vi "SSC DAQmx Read TEDS.vi"(0 "DAQmx SSC in":T2[](array[typedef]), 11 "error in":errorcluster) -> (4 "DAQmx SSC out":T2[](array[typedef]), 6 "SSC TEDS BitStream":T1[][](array[typedef]), 15 "error out":errorcluster)   [LabVIEW 2020]
doc: "Reads the TEDS bitstream in the order of SSC."
uses:
  Pin Map/SSC DAQmx.ctl
  Typedefs/SSC TEDS Bitstream.ctl
  <resource>/objmgr/daqmx.rc
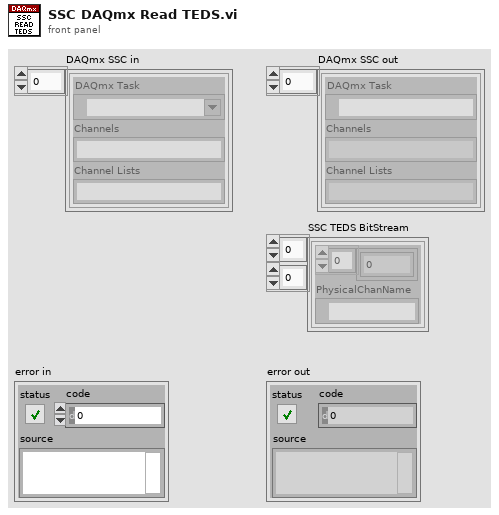
[diagram p1: front panel]
types:
  T1 = typedef "SSC TEDS Bitstream.ctl" = cluster{"TEDS BitStream":u8[], "PhysicalChanName":tag}
  T2 = typedef "SSC DAQmx.ctl" = cluster{"DAQmx Task ":refnum<k21>, "Channels":string, "Channel Lists":string}
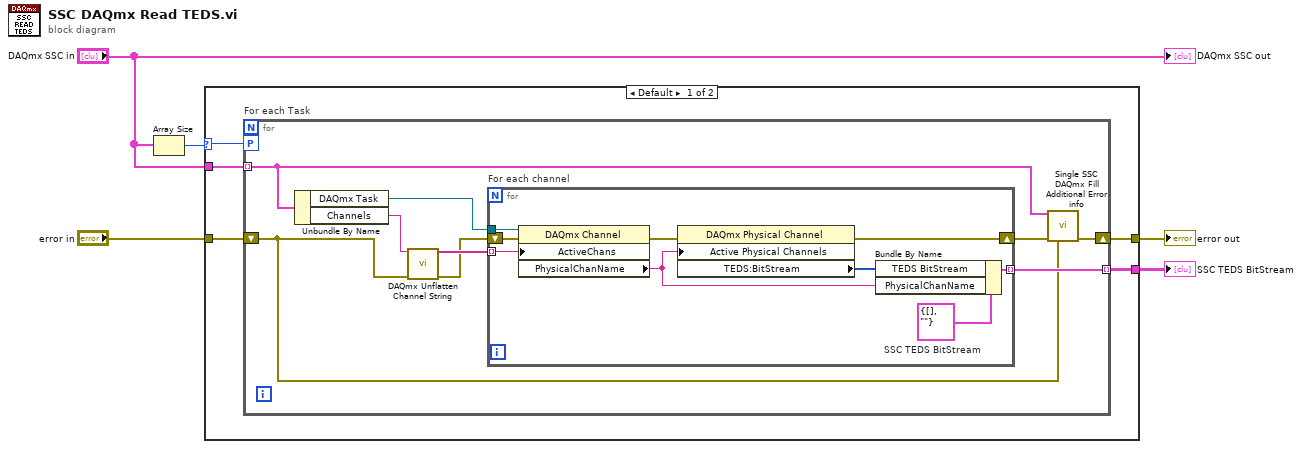
[diagram p0: block diagram]
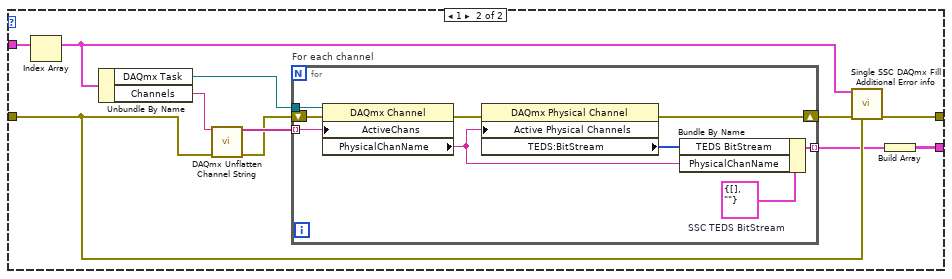
[diagram p2: hidden frame]
diagram:
  n1 = Array Size(array="DAQmx SSC in") -> (size(s)=w3:i32)
  n2 = case shown="Default" w3 {
    selector: w3 -> [w8 _]
    tunnel: [w10 w39] -> w5
    tunnel: "error in" -> [w9 w38]
    tunnel: "DAQmx SSC in" -> [w7 w37]
    tunnel: [w6 w29] -> w1
    frame Default {
      n3 = for "For each Task" {
        tunnel: w7 -> [w18] mode=indexing
        workers-P: w8 -> [_]
        shift-right: [w19] -> w10
        shift-left: w9 -> [w12]
        tunnel: [w15] -> w6 mode=indexing
        n4 = Unbundle By Name(w18) -> ("DAQmx Task"=w16:refnum<k21>, "Channels"=w14:string)
        n5 = call <vilib>:"DAQmx Unflatten Channel String.vi"("names in"=w14, "error in"=w12) -> ("names out"=w13:string[], "error out"=w11:errorcluster)  [unwired: 12 in]
        n6 = for "For each channel" {
          shift-right: [w28] -> w17
          shift-left: w11 -> [w27]
          tunnel: w16 -> [w25]
          tunnel: w13 -> [w24] mode=indexing
          tunnel: [w22] -> w15 mode=indexing
          w23 = T1 {"TEDS BitStream"=[], "PhysicalChanName"=""}  # SSC TEDS BitStream
          n7 = property class="DAQmx Channel"(reference=w25, error in=w27, "ActiveChans"=w24) -> (error out=w26:errorcluster, "PhysicalChanName"=w20:tag)  [unwired: 1 out]
          n8 = property class="DAQmx Physical Channel"(error in=w26, "Active Physical Channels"=w20) -> (error out=w28:errorcluster, "TEDS:BitStream"=w21:u8[])  [unwired: 1 in, 1 out]
          n9 = Bundle By Name(cluster=w23, "TEDS BitStream"=w21, "PhysicalChanName"=w20) -> (w22:T1)
        }
        n10 = call "Single SSC DAQmx Fill Additional Error info.vi"("DAQmx SSC in"=w18, "error in"=w17, "previous error in"=w12) -> ("error out"=w19:errorcluster)  [unwired: 12 in]
      }
    }
    frame 1 {
      n11 = Index Array(array=w37) -> (element=w30:T2)  [unwired: 1 in]
      n12 = Unbundle By Name(w30) -> ("DAQmx Task"=w34:refnum<k21>, "Channels"=w33:string)
      n13 = call <vilib>:"DAQmx Unflatten Channel String.vi"("names in"=w33, "error in"=w38) -> ("names out"=w32:string[], "error out"=w31:errorcluster)  [unwired: 12 in]
      n14 = for "For each channel" {
        shift-right: [w48] -> w35
        shift-left: w31 -> [w47]
        tunnel: w34 -> [w45]
        tunnel: w32 -> [w44] mode=indexing
        tunnel: [w42] -> w36 mode=indexing
        w43 = T1 {"TEDS BitStream"=[], "PhysicalChanName"=""}  # SSC TEDS BitStream
        n15 = property class="DAQmx Channel"(reference=w45, error in=w47, "ActiveChans"=w44) -> (error out=w46:errorcluster, "PhysicalChanName"=w40:tag)  [unwired: 1 out]
        n16 = property class="DAQmx Physical Channel"(error in=w46, "Active Physical Channels"=w40) -> (error out=w48:errorcluster, "TEDS:BitStream"=w41:u8[])  [unwired: 1 in, 1 out]
        n17 = Bundle By Name(cluster=w43, "TEDS BitStream"=w41, "PhysicalChanName"=w40) -> (w42:T1)
      }
      n18 = call "Single SSC DAQmx Fill Additional Error info.vi"("DAQmx SSC in"=w30, "error in"=w35, "previous error in"=w38) -> ("error out"=w39:errorcluster)  [unwired: 12 in]
      n19 = Build Array(w36) -> (w29:T1[][])
    }
  }
  "error out" <- w5
  "SSC TEDS BitStream" <- w1
  "DAQmx SSC out" <- "DAQmx SSC in"
